vi "Boolean Array To Number.vi"() -> ()   [LabVIEW 2021]
panel:
  out "error out":errorcluster
  out "data string":string
  in  "stop":bool
  out "number":u32
  in  "AO":bool
  in  "AI":bool
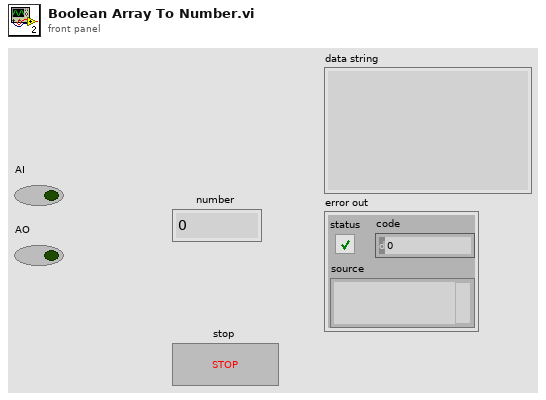
[diagram p1: front panel]
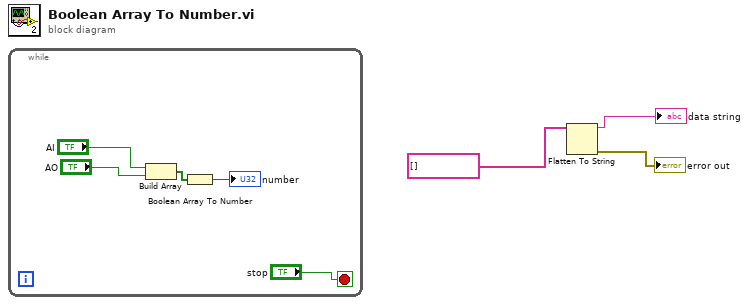
[diagram p0: block diagram]
diagram:
  n1 = while {
    stop <- "stop" stop-if-true
    n2 = Build Array("AI", "AO") -> (w6:bool[])
    n3 = Boolean Array To Number(Boolean array=w6) -> (number=→"number":u32)
  }
  n4 = Flatten To String(anything=tag[] [] ("AI Physical Channels")) -> (data string=→"data string":string, error out=→"error out":errorcluster)  [unwired: 3 in, 1 out]
